vi "BUFMNGR_optimize.vi"(9 "size":u64, 10 "optimize":string) -> ()   [LabVIEW 2016]
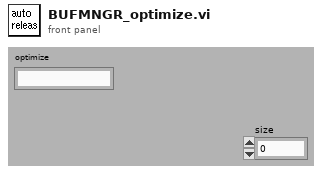
[diagram p1: front panel]
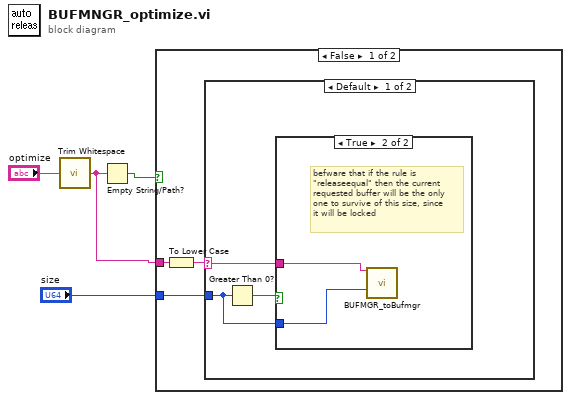
[diagram p0: block diagram]
diagram:
  n1 = call <vilib>:"Trim Whitespace.vi"("string"="optimize") -> ("trimmed string"=w2:string)  [unwired: 1 in]
  n2 = Empty String/Path?(string/path=w2) -> (empty?=w3:bool)
  n3 = case shown="False" w3 {
    tunnel: w2 -> [w6 _]
    tunnel: "size" -> [w7 _]
    frame False {
      n4 = To Lower Case(string=w6) -> (all lower case string=w5:string)
      n5 = case shown="Default" w5 {
        selector: w5 -> [w9 _]
        tunnel: w7 -> [w8 _]
        frame Default {
          n6 = Greater Than 0?(x=w8) -> (x > 0?=w10:bool)
          n7 = case shown="True" w10 {
            tunnel: w9 -> [_ w11]
            tunnel: w8 -> [_ w12]
            frame False {
            }
            frame True {
              # "befware that if the rule is\n\"releaseequal\" then the current\nrequested buffer will be the only\none to survive of this size, since\nit will be locked"
              n8 = call "BUFMGR_toBufmgr.vi"("command"=w11, "bufsize"=w12) -> ()  [unwired: 6 in, 8 out]
            }
          }
        }
        frame "false", "no", "none", "off" {
        }
      }
    }
    frame True {
    }
  }
